vi "Actor Core.vi"(8 "error in":errorcluster, 11 "Guardar TextoPlano in":refnum<class "Guardar TextoPlano.lvclass">) -> (0 "error out":errorcluster, 3 "Actor out":refnum<class "Actor.lvclass">)   [LabVIEW 2020, in "Guardar TextoPlano.lvlib" / "Guardar TextoPlano.lvclass"]
doc: "(<B>Filename</B>: Actor Framework.lvlib:Actor.lvclass:Actor Core.vi)\n\nReceives messages to the actor, reacts to them, and initiates any error handling that may shut the actor down.\n\nDescendant classes may override this VI to append parallel tasks for the actor to complete while it handles messages. Overrides use the Call Parent Class Method node."
uses:
  Guardar TextoPlano.lvclass
  <vilib>/ActorFramework/Actor/Actor.lvclass
  Guardar TextoPlano.lvclass/Guardar TextoPlano.ctl
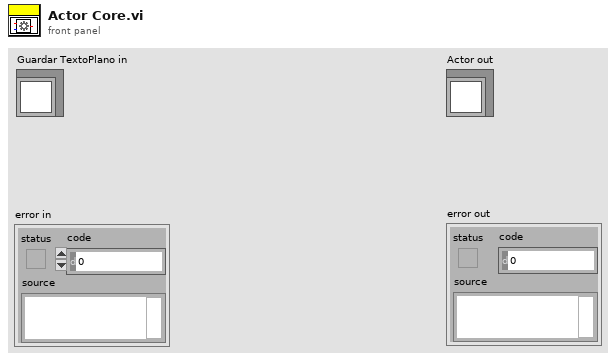
[diagram p1: front panel]
types:
  T1 = cluster{"Path":path, "Proviene de?":enum16{"Contador", "Generador funciones"}, "Dato":string}
  T2 = cluster{"Path Event":refnum<user-event>, "Save? Event":refnum<user-event>, "Exit Event":refnum<user-event>, "Datos Event":refnum<user-event>, "Provienede? EVENT":refnum<user-event>}
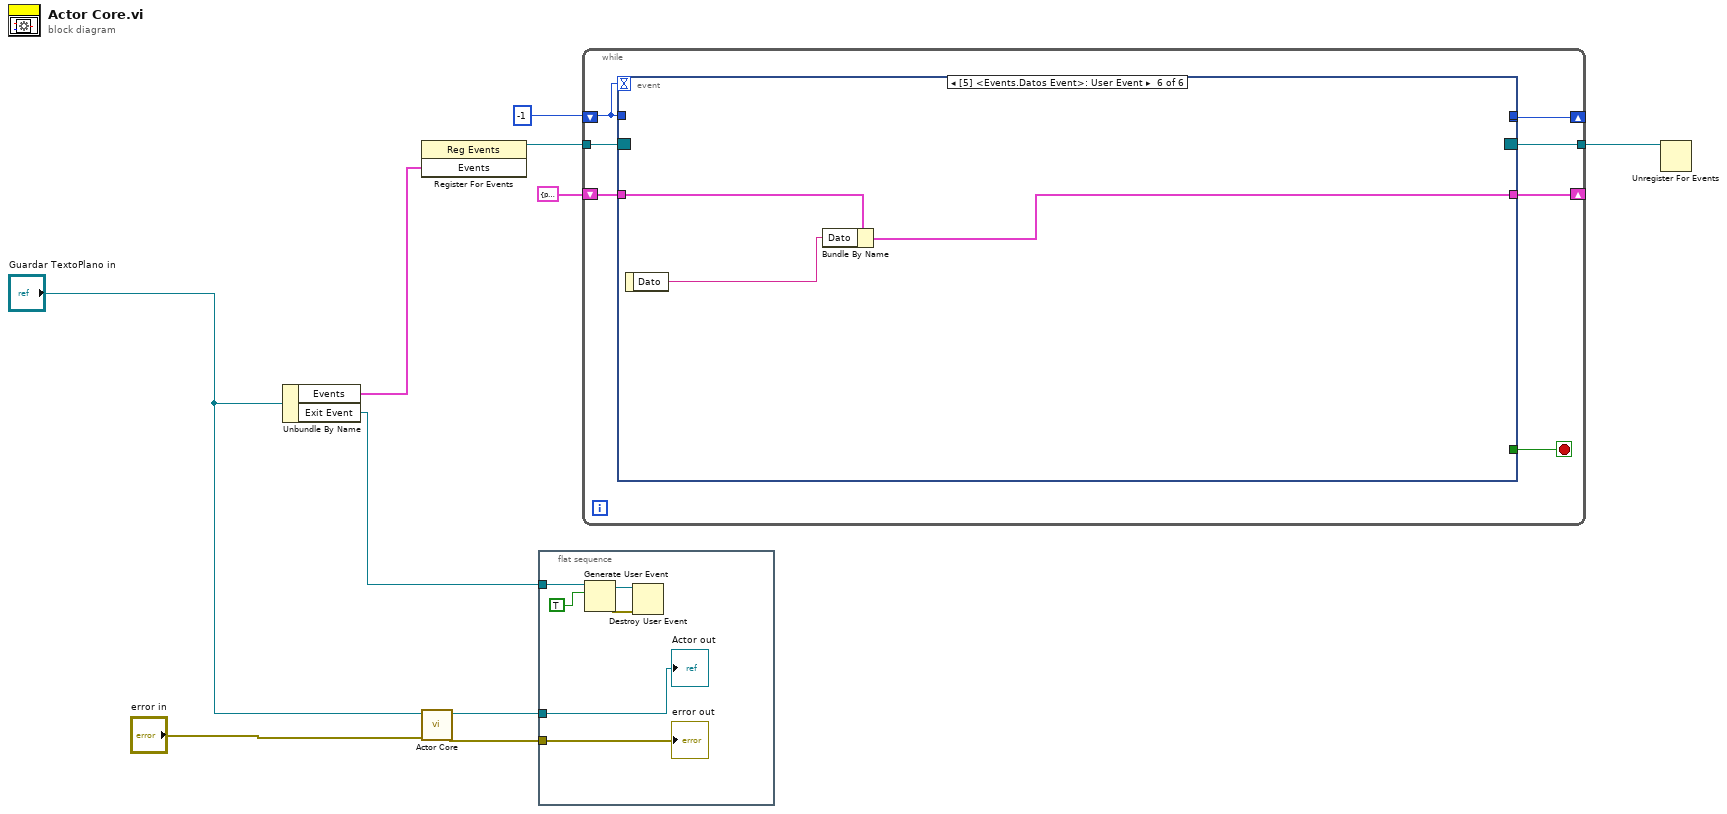
[diagram p0: block diagram]
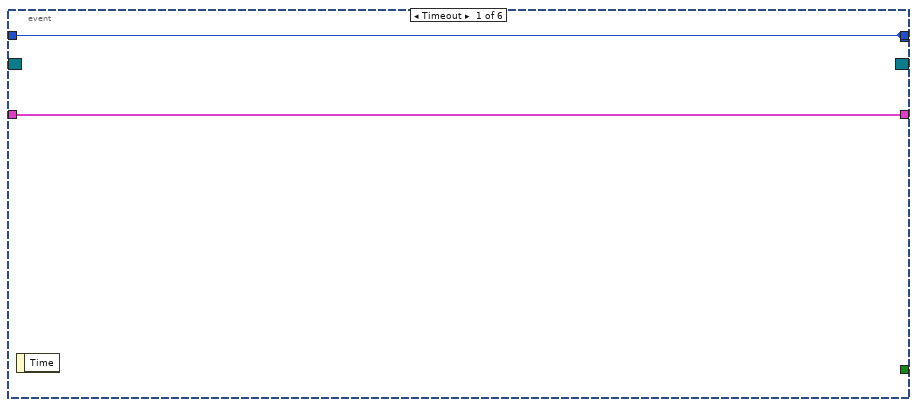
[diagram p2: hidden frame]
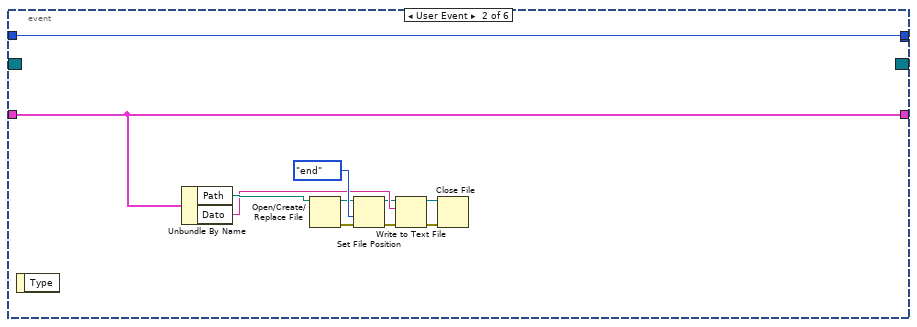
[diagram p3: hidden frame]
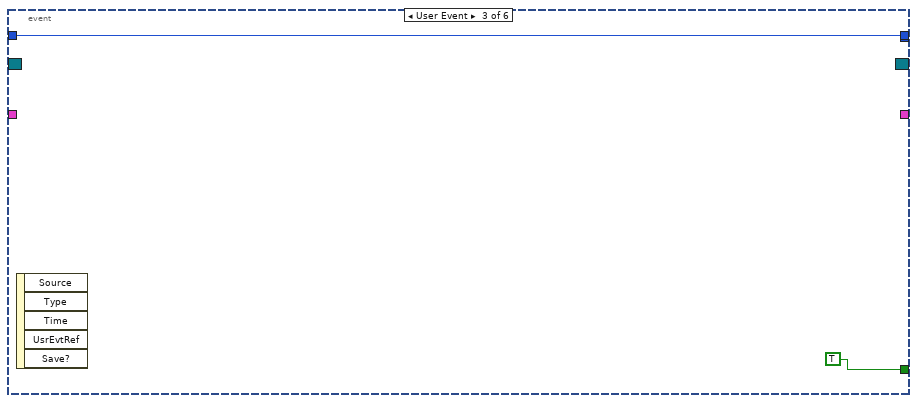
[diagram p4: hidden frame]
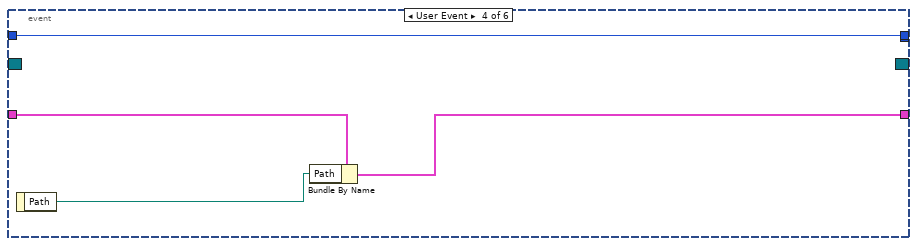
[diagram p5: hidden frame]
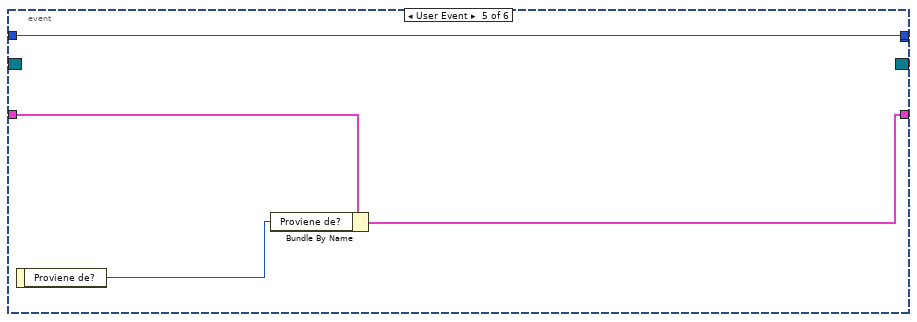
[diagram p6: hidden frame]
diagram:
  n1 = Unbundle By Name("Guardar TextoPlano in") -> ("Events"=w5:T2, "Exit Event"=w6:refnum<user-event>)
  n2 = register-events(w5) -> (reference out=w3:refnum<event-registration>)  [unwired: 2 in, 1 out]
  n3 = call-parent "Actor Core.vi"("error in"="error in", "Actor in"="Guardar TextoPlano in") -> ("error out"=w10:errorcluster, "Actor out"=w9:refnum<class "Actor.lvclass">)  [unwired: 8 in]
  n4 = flat-sequence {
    tunnel: w10 -> [w16]
    tunnel: w9 -> [w15]
    tunnel: w6 -> [w12]
    frame #0 {
      n5 = Generate User Event(user event=w12, event data cluster=TRUE ("event data")) -> (user event out=w14:refnum<user-event>, error out=w13:errorcluster)  [unwired: 2 in]
      n6 = Destroy User Event(user event=w14, error in=w13) -> ()  [unwired: 1 out]
      "error out" <- w16
      "Actor out" <- w15
    }
  }
  n7 = while {
    shift-right: [w23] -> _
    shift-left: -1 -> [w22]
    tunnel: w3 -> [w21]
    shift-right: [w19] -> _
    shift-left: T1 {"Path"=path "", "Proviene de?"=enum."Contador", "Dato"=""} -> [w20]
    tunnel: [w18] -> w1
    stop <- w17 stop-if-true
    n8 = event shown="[5] <Events.Datos Event>: User Event" {
      selector: w21 -> [_ _ _ _ _ _]
      dyn-events: [_ _ _ _ _ _] -> w18
      timeout: w22 -> [_ _ _ _ _ _]
      tunnel: w22 -> [w25 w26 w37 w42 w43 _]
      tunnel: [w25 w26 w37 w42 w43 _] -> w23
      tunnel: [w25 _ _ _ _ _] -> _
      tunnel: [w24 w27 _ w39 w45 w47] -> w19
      tunnel: w20 -> [w24 w27 _ w41 w46 w49]
      tunnel: [_ _ TRUE _ _ _] -> w17
      event Timeout {
        n9 = event-data() -> ()  [unwired: 1 in, 1 out]
      }
      event User Event {
        n10 = event-data() -> ()  [unwired: 1 in, 1 out]
        n11 = Unbundle By Name(w27) -> ("Path"=w35:path, "Dato"=w34:string)
        n12 = Open/Create/Replace File(file path (use dialog)=w35) -> (refnum out=w33:refnum<file>, error out=w31:errorcluster)  [unwired: 5 in, 1 out]
        n13 = Set File Position(refnum=w33, from (0:start)=enum16{"start", "end", "current"}."end", error in=w31) -> (refnum out=w32:refnum<file>, error out=w30:errorcluster)  [unwired: 1 in]
        n14 = Write to Text File(file (use dialog)=w32, text=w34, error in=w30) -> (refnum out=w29:refnum<file>, error out=w28:errorcluster)  [unwired: 1 in, 1 out]
        n15 = Close File(refnum=w29, error in=w28) -> ()  [unwired: 2 out]
      }
      event User Event {
        n16 = event-data() -> ()  [unwired: 1 in, 5 out]
      }
      event User Event {
        n17 = event-data() -> ("Path"=w40:path)  [unwired: 1 in]
        n18 = Bundle By Name(cluster=w41, "Path"=w40) -> (w39:T1)
      }
      event User Event {
        n19 = event-data() -> ("Proviene de?"=w44:enum16{"Contador", "Generador funciones"})  [unwired: 1 in]
        n20 = Bundle By Name(cluster=w46, "Proviene de?"=w44) -> (w45:T1)
      }
      event User Event {
        n21 = event-data() -> ("Dato"=w48:string)  [unwired: 1 in]
        n22 = Bundle By Name(cluster=w49, "Dato"=w48) -> (w47:T1)
      }
    }
  }
  n23 = Unregister For Events(event registration refnum=w1) -> ()  [unwired: 1 in, 1 out]
